vi "Initialize Parallel Events.vi"(8 "error in (no error)":errorcluster, 11 "CIFPluginManager in":refnum<class "CIFPluginManager.lvclass">) -> (0 "error out":errorcluster, 3 "CIFPluginManager out":refnum<class "CIFPluginManager.lvclass">)   [LabVIEW 2021, in "CIFPluginManager.lvclass"]
uses:
  CIFPluginManager.lvclass
  typedef/Discover Command.ctl
  typedef/Plugin Load Command.ctl
  Common/typedef/Loader Type.ctl
  typedef/Loader Load Command.ctl
  CIFPluginManager.lvclass/CIFPluginManager.ctl
  Common/Manager Common.lvlib
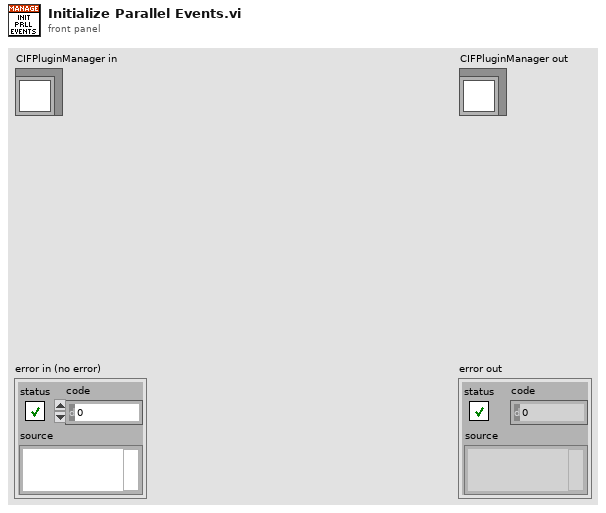
[diagram p1: front panel]
types:
  T1 = typedef "CIFPluginManager.lvclass/Discover Command.ctl" = cluster{"Loader Name":string, "Update Metadata":bool}
  T2 = typedef "CIFPluginManager.lvclass/Plugin Load Command.ctl" = cluster{"Plugin Name":string, "Plugin Path":string, "Loader Name":string, "Loader Type":T3}
  T3 = typedef "Manager Common.lvlib/Loader Type.ctl" = enum16{"LabVIEW"}
  T4 = typedef "CIFPluginManager.lvclass/Loader Load Command.ctl" = cluster{"Loader Type":T3, "Loader Name":string}
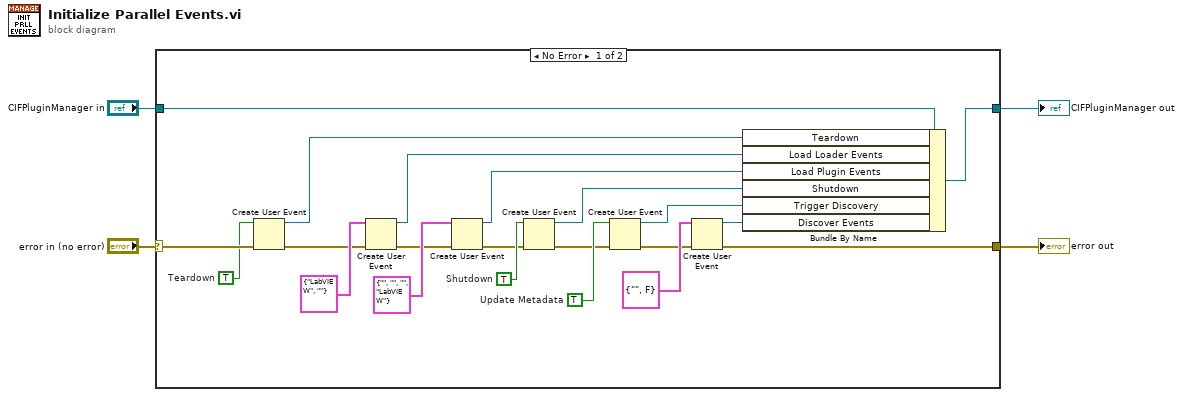
[diagram p0: block diagram]
diagram:
  n1 = case shown="No Error" "error in (no error)" {
    selector: "error in (no error)" -> [w8 w27]
    tunnel: [w9 w27] -> w3
    tunnel: [w24 w26] -> w1
    tunnel: "CIFPluginManager in" -> [w25 w26]
    frame No Error {
      w6 = TRUE  # Teardown
      w20 = TRUE  # Shutdown
      w23 = TRUE  # Update Metadata
      n2 = Create User Event(user event datatype=w6, error in=w8) -> (user event=w5:refnum<user-event>, error out=w7:errorcluster)
      n3 = Create User Event(user event datatype=T4 {"Loader Type"=enum."LabVIEW", "Loader Name"=""} ("Launcher Load Info"), error in=w7) -> (user event=w17:refnum<user-event>, error out=w13:errorcluster)
      n4 = Create User Event(user event datatype=T2 {"Plugin Name"="", "Plugin Path"="", "Loader Name"="", "Loader Type"=enum."LabVIEW"} ("Plugin Load Info"), error in=w13) -> (user event=w15:refnum<user-event>, error out=w14:errorcluster)
      n5 = Create User Event(user event datatype=w20, error in=w14) -> (user event=w19:refnum<user-event>, error out=w21:errorcluster)
      n6 = Create User Event(user event datatype=w23, error in=w21) -> (user event=w22:refnum<user-event>, error out=w10:errorcluster)
      n7 = Create User Event(user event datatype=T1 {"Loader Name"="", "Update Metadata"=FALSE} ("Discover Command"), error in=w10) -> (user event=w11:refnum<user-event>, error out=w9:errorcluster)
      n8 = Bundle By Name(cluster=w25, "Teardown"=w5, "Load Loader Events"=w17, "Load Plugin Events"=w15, "Shutdown"=w19, "Trigger Discovery"=w22, "Discover Events"=w11) -> (w24:refnum<class "CIFPluginManager.lvclass">)
    }
    frame Error {
    }
  }
  "error out" <- w3
  "CIFPluginManager out" <- w1
